vi "Func-엑셀 데이터를 그래프로 출력.vi"() -> ()   [LabVIEW 2015] (continued)
\n1158.26\n1158.28\n1158.3\n1158.31\n1158.33\n1158.34\n1158.36\n1158.38\n1158.39\n1158.41\n1158.43\n1158.44\n1158.46\n1158.48\n1158.49\n1158.51\n1158.53\n1158.55\n1158.56\n1158.58\n1158.59\n1158.61\n1158.63\n1158.65\n1158.66\n1158.68\n1158.69\n1158.71\n1158.73\n1158.74\n1158.76\n1158.78\n1158.8\n1158.81\n1158.83\n1158.84\n1158.86\n1158.88\n1158.89\n1158.91\n1158.93\n1158.94\n1158.96\n1158.98\n1159\n1159.01\n1159.03\n1159.04\n1159.06\n1159.08\n1159.09\n1159.11\n1159.13\n1159.15\n1159.16\n1159.18\n1159.19\n1159.21\n1159.23\n1159.25\n1159.26\n1159.28\n1159.29\n1159.31\n1159.33\n1159.35\n1159.36\n1159.38\n1159.39\n1159.41\n1159.43\n1159.44\n1159.46\n1159.48\n1159.5\n1159.51\n1159.53\n1159.54\n1159.56\n1159.58\n1159.59\n1159.61\n1159.63\n1159.64\n1159.66\n1159.68\n1159.69\n1159.71\n1159.73\n1159.74\n1159.76\n1159.78\n1159.79\n1159.81\n1159.83\n1159.84\n1159.86\n1159.88\n1159.89\n1159.91\n1159.93\n1159.94\n1159.96\n1159.98\n1159.99\n1160.01\n1160.03\n1160.04\n1160.06\n1160.08\n1160.09\n1160.11\n1160.13\n1160.14\n1160.16\n1160.18\n1160.19\n1160.21\n1160.23\n1160.24\n1160.26\n1160.28\n1160.29\n1160.31\n1160.33\n1160.34\n1160.36\n1160.38\n1160.39\n1160.41\n1160.43\n1160.44\n1160.46\n1160.48\n1160.49\n1160.51\n1160.53\n1160.54\n1160.56\n1160.58\n1160.59\n1160.61\n1160.63\n1160.64\n1160.66\n1160.68\n1160.69\n1160.71\n1160.73\n1160.74\n1160.76\n1160.78\n1160.79\n1160.81\n1160.83\n1160.84\n1160.86\n1160.88\n1160.89\n1160.91\n1160.93\n1160.94\n1160.96\n1160.98\n1160.99\n1161.01\n1161.03\n1161.04\n1161.06\n1161.08\n1161.09\n1161.11\n1161.13\n1161.14\n1161.16\n1161.18\n1161.19\n1161.21\n1161.23\n1161.24\n1161.26\n1161.28\n1161.3\n1161.31\n1161.33\n1161.34\n1161.36\n1161.38\n1161.39\n1161.41\n1161.43\n1161.44\n1161.46\n1161.48\n1161.49\n1161.51\n1161.53\n1161.55\n1161.56\n1161.58\n1161.59\n1161.61\n1161.63\n1161.65\n1161.66\n1161.68\n1161.69\n1161.71\n1161.73\n1161.75\n1161.76\n1161.78\n1161.79\n1161.81\n1161.83\n1161.84\n1161.86\n1161.88\n1161.9\n1161.91\n1161.93\n1161.94\n1161.96\n1161.98\n1162\n1162.01\n1162.03\n1162.04\n1162.06\n1162.08\n1162.1\n1162.11\n1162.13\n1162.14\n1162.16\n1162.18\n1162.19\n1162.21\n1162.23\n1162.25\n1162.26\n1162.28\n1162.29\n1162.31\n1162.33\n1162.35\n1162.36\n1162.38\n1162.39\n1162.41\n1162.43\n1162.45\n1162.46\n1162.48\n1162.49\n1162.51\n1162.53\n1162.55\n1162.56\n1162.58\n1162.59\n1162.61\n1162.63\n1162.64\n1162.66\n1162.68\n1162.7\n1162.71\n1162.73\n1162.74\n1162.76\n1162.78\n1162.79\n1162.81\n1162.83\n1162.84\n1162.86\n1162.88\n1162.89\n1162.91\n1162.93\n1162.95\n1162.96\n1162.98\n1162.99\n1163.01\n1180.53\n1180.71\n1180.87\n1181.04\n1181.21\n1181.37\n1181.55\n1181.71\n1181.88\n1182.05\n1182.21\n1182.38\n1182.55\n1182.71\n1182.88\n1183.05\n1183.21\n1183.38\n1183.55\n1183.72\n1183.88\n1184.05\n1184.21\n1184.38\n1184.55\n1184.71\n1184.88\n1185.05\n1185.21\n1185.38\n1185.55\n1185.71\n1185.88\n1186.06\n1186.22\n1186.39\n1186.56\n1186.73\n1186.9\n1187.07\n1187.23\n1187.4\n1187.56\n1187.73\n1187.9\n1188.06\n1188.23\n1188.4\n1188.56\n1188.73\n1188.9\n1189.07\n1189.24\n1189.41\n1189.57\n1189.74\n1189.91\n1190.07\n1190.24\n1190.41\n1190.57\n1190.74\n1190.91\n1191.07\n1191.24\n1191.41\n1191.57\n1191.74\n1191.91\n1192.07\n1192.24\n1192.41\n1192.57\n1192.74\n1192.91\n1193.07\n1193.24\n1193.41\n1193.57\n1193.74\n1193.91\n1194.07\n1194.24\n1194.41\n1194.57\n1194.74\n1194.91\n1195.07\n1195.24\n1195.41\n1195.57\n1195.74\n1195.91\n1196.07\n1196.24\n1196.41\n1196.57\n1196.74\n1196.91\n1197.07\n1197.24\n1197.41\n1197.58\n1197.75\n1197.91\n1198.08\n1198.25\n1198.42\n1198.58\n1198.75\n1198.91\n1199.08\n1199.25\n1199.41\n1199.58\n1199.75\n1199.91\n1200.08\n1200.25\n1200.41\n1200.58\n1200.75\n1200.91\n1201.08\n1201.25\n1201.42\n1201.58\n1201.75\n1201.92\n1202.09\n1202.26\n1202.42\n1202.59\n1202.76\n1202.92\n1203.09\n1203.26\n1203.42\n1203.6\n1203.76\n1203.93\n1204.1\n1204.27\n1204.43\n1204.6\n1204.77\n1204.93\n1205.1\n1205.26\n1205.43\n1205.6\n1205.76\n1205.93\n1206.1\n1206.26\n1206.43\n1206.6\n1206.76\n1206.93\n1207.1\n1207.26\n1207.43\n1207.6\n1207.76\n1207.93\n1208.1\n1208.26\n1208.43\n1208.6\n1208.76\n1208.93\n1209.1\n1209.26\n1209.43\n1209.6\n1209.76\n1209.93\n1210.1\n1210.26\n1210.43\n1210.6\n1210.76\n1210.93\n1211.1\n1211.26\n1211.43\n1211.6\n1211.76\n1211.93\n1212.11\n1212.28\n1212.45\n1212.61\n1212.78\n1212.95\n1213.12\n1213.28\n1213.45\n1213.61\n1213.78\n1213.95\n1214.11\n1214.28\n1214.45\n1214.61\n1214.79\n1214.96\n1215.12\n1215.29\n1215.46\n1215.62\n1215.79\n1215.96\n1216.12\n1216.29\n1216.46\n1216.62\n1216.79\n1216.96\n1217.13\n1217.3\n1217.47\n1217.64\n1217.81\n1217.97\n1218.14\n1218.31\n1218.48\n1218.65\n1218.81\n1218.98\n1219.15\n1219.32\n1219.48\n1219.65\n1219.81\n1219.98\n1220.15\n1220.31\n1220.48\n1220.65\n1220.81\n1220.99\n1221.17\n1221.33\n1221.5\n1221.66\n1221.83\n1222.01\n1222.18\n1222.35\n1222.51\n1222.68\n1222.85\n1223.02\n1223.18\n1223.35\n1223.51\n1223.68\n1223.85\n1224.01\n1224.17\n1224.18\n1224.19\n1224.21\n1224.23\n1224.24\n1224.26\n1224.28\n1224.29\n1224.31\n1224.33\n1224.34\n1224.36\n1224.38\n1224.39\n1224.41\n1224.43\n1224.44\n1224.46\n1224.48\n1224.49\n1224.51\n1224.53\n1224.54\n1224.56\n1224.58\n1224.59\n1224.61\n1224.63\n1224.64\n1224.66\n1224.68\n1224.69\n1224.71\n1224.73\n1224.74\n1224.76\n1224.78\n1224.79\n1224.81\n1224.83\n1224.84\n1224.86\n1224.88\n1224.89\n1224.91\n1224.93\n1224.94\n1224.96\n1224.98\n1224.99\n1225.01\n1225.03\n1225.05\n1225.06\n1225.08\n1225.09\n1225.11\n1225.13\n1225.14\n1225.16\n1225.18\n1225.19\n1225.21\n1225.23\n1225.24\n1225.26\n1225.28\n1225.29\n1225.31\n1225.33\n1225.34\n1225.36\n1225.38\n1225.39\n1225.41\n1225.43\n1225.44\n1225.46\n1225.48\n1225.49\n1225.51\n1225.53\n1225.54\n1225.56\n1225.58\n1225.59\n1225.61\n1225.63\n1225.64\n1225.66\n1225.68\n1225.69\n1225.71\n1225.73\n1225.74\n1225.76\n1225.78\n1225.79\n1225.81\n1225.83\n1225.85\n1225.86\n1225.88\n1225.89\n1225.91\n1225.93\n1225.94\n1225.96\n1225.98\n1225.99\n1226.01\n1226.03\n1226.04\n1226.06\n1226.08\n1226.1\n1226.11\n1226.13\n1226.14\n1226.16\n1226.18\n1226.2\n1226.21\n1226.23\n1226.25\n1226.26\n1226.28\n1226.3\n1226.31\n1226.33\n1226.34\n1226.36\n1226.38\n1226.39\n1226.41\n1226.43\n1226.44\n1226.46\n1226.48\n1226.49\n1226.51\n1226.53\n1226.55\n1226.56\n1226.58\n1226.59\n1226.61\n1226.63\n1226.64\n1226.66\n1226.68\n1226.7\n1226.71\n1226.73\n1226.74\n1226.76\n1226.78\n1226.79\n1226.81\n1226.83\n1226.84\n1226.86\n1226.88\n1226.9\n1226.91\n1226.93\n1226.94\n1226.96\n1226.98\n1226.99\n1227.01\n1227.03\n1227.04\n1227.06\n1227.08\n1227.09\n1227.11\n1227.13\n1227.14\n1227.16\n1227.18\n1227.19\n1227.21\n1227.23\n1227.24\n1227.26\n1227.28\n1227.29\n1227.31\n1227.33\n1227.34\n1227.36\n1227.38\n1227.4\n1227.41\n1227.43\n1227.44\n1227.46\n1227.48\n1227.49\n1227.51\n1227.53\n1227.54\n1227.56\n1227.58\n1227.59\n1227.61\n1227.63\n1227.64\n1227.66\n1227.68\n1227.69\n1227.71\n1227.73\n1227.74\n1227.76\n1227.78\n1227.8\n1227.81\n1227.83\n1227.84\n1227.86\n1227.88\n1227.89\n1227.91\n1227.93\n1227.94\n1227.96\n1227.98\n1227.99\n1228.01\n1228.03\n1228.04\n1228.06\n1228.08\n1228.09\n1228.11\n1228.13\n1228.14\n1228.16\n1228.18\n1228.19\n1228.21\n1228.23\n1228.24\n1228.26\n1228.28\n1228.29\n1228.31\n1228.33\n1228.34\n1228.36\n1228.38\n1228.39\n1228.41\n1228.43\n1228.44\n1228.46\n1228.48\n1228.49\n1228.51\n1228.53\n1228.54\n1228.56\n1228.58\n1228.6\n1228.61\n1228.63\n1228.64\n1228.66\n1228.68\n1228.69\n1228.71\n1228.73\n1228.74\n1228.76\n1228.78\n1228.79\n1228.81\n1228.83\n1228.85\n1228.86\n1228.88\n1228.89\n1228.91\n1228.93\n1228.95\n1228.96\n1228.98\n1229\n1229.01\n1229.03\n1229.04\n1229.06\n1229.08\n1229.09\n1229.11\n1229.13\n1229.14\n1229.16\n1229.18\n1229.2\n1229.21\n1229.23\n1229.24\n1229.26\n1229.28\n1229.3\n1229.31\n1229.33\n1229.34\n1229.36\n1229.38\n1229.4\n1229.41\n1229.43\n1229.44\n1229.46\n1229.48\n1229.49\n1229.51\n1229.53\n1229.55\n1229.56\n1229.58\n1229.59\n1229.61\n1229.63\n1229.64\n1229.66\n1229.68\n1229.69\n1229.71\n1229.73\n1229.74\n1229.76\n1229.78\n1229.79\n1229.81\n1229.83\n1229.84\n1229.86\n1229.88\n1229.89\n1229.91\n1229.93\n1229.94\n1229.96\n1229.98\n1229.99\n1230.01\n1230.03\n1230.04\n1230.06\n1230.08\n1230.09\n1230.11\n1230.13\n1230.14\n1230.16\n1230.18\n1230.19\n1230.21\n1230.23\n1230.24\n1230.26\n1230.28\n1230.29\n1230.31\n1230.33\n1230.34\n1230.36\n1230.38\n1230.39\n1230.41\n1230.43\n1230.44\n1230.46\n1230.48\n1230.49\n1230.51\n1230.53\n1230.54\n1230.56\n1230.58\n1230.59\n1230.61\n1230.63\n1230.64\n1230.66\n1230.68\n1230.69\n1230.71\n1230.73\n1230.74\n1230.76\n1230.78\n1230.79\n1230.81\n1230.83\n1230.84\n1230.86\n1230.88\n1230.89\n1230.91\n1230.93\n1230.94\n1230.96\n1230.98\n1230.99\n1231.01\n1231.03\n1231.04\n1231.06\n1231.08\n1231.09\n1231.11\n1231.13\n1231.14\n1231.16\n1231.18\n1231.19\n1231.21\n1231.23\n1231.24\n1231.26\n1231.28\n1231.29\n1231.31\n1231.33\n1231.34\n1231.36\n1231.38\n1231.39\n1231.41\n1231.43\n1231.44\n1231.46\n1231.48\n1231.49\n1231.51\n1231.53\n1231.54\n1231.56\n1231.58\n1231.6\n1231.61\n1231.63\n1231.64\n1231.66\n1231.68\n1231.69\n1231.71\n1231.73\n1231.74\n1231.76\n1231.78\n1231.79\n1231.81\n1231.83\n1231.84\n1231.86\n1231.88\n1231.89\n1231.91\n1231.93\n1231.95\n1231.96\n1231.98\n1231.99\n1232.01\n1232.03\n1232.05\n1232.06\n1232.08\n1232.09\n1232.11\n1232.13\n1232.14\n1232.16\n1232.18\n1232.2\n1232.21\n1232.23\n1232.24\n1232.26\n1232.28\n1232.3\n1232.31\n1232.33\n1232.34\n1232.36\n1232.38\n1232.4\n1232.41\n1232.43\n1232.44\n1232.46\n1232.48\n1232.49\n1232.51\n1232.53\n1232.54\n1232.56\n1232.58\n1232.59\n1232.61\n1232.63\n1232.64\n1232.66\n1232.68\n1232.69\n1232.71\n1232.73\n1232.74\n1232.76\n1232.78\n1232.79\n1232.81\n1232.83\n1232.84\n1232.86\n1232.88\n1232.89\n1232.91\n1232.93\n1232.94\n1232.96\n1232.98\n1232.99\n1233.01\n1233.03\n1233.04\n1233.06\n1233.08\n1233.09\n1233.11\n1233.13\n1233.14\n1233.16\n1233.18\n1233.19\n1233.21\n1233.23\n1233.24\n1233.26\n1233.28\n1233.29\n1233.31\n1233.33\n1233.34\n1233.36\n1233.38\n1233.39\n1233.41\n1233.43\n1233.44\n1233.46\n1233.48\n1233.49\n1233.51\n1233.53\n1233.54\n1233.56\n1233.58\n1233.59\n1233.61\n1233.63\n1233.64\n1233.66\n1233.68\n1233.69\n1233.71\n1233.73\n1233.74\n1233.76\n1233.78\n1233.79\n1233.81\n1233.83\n1233.84\n1233.86\n1233.88\n1233.89\n1233.91\n1233.93\n1233.94\n1233.96\n1233.98\n1233.99\n1234.01\n1234.03\n1234.04\n1234.06\n1234.08\n1234.09\n1234.11\n1234.13\n1234.14\n1234.16\n1234.18\n1234.19\n1234.21\n1234.23\n1234.24\n1234.26\n1234.28\n1234.29\n1234.31\n1234.33\n1234.35\n1234.36\n1234.38\n1234.39\n1234.41\n1234.43\n1234.44\n1234.46\n1234.48\n1234.49\n1234.51\n1234.53\n1234.54\n1234.56\n1234.58\n1234.59\n1234.61\n1234.63\n1234.64\n1234.66\n1234.68\n1234.7\n1234.71\n1234.73\n1234.74\n1234.76\n1234.78\n1234.8\n1234.81\n1234.83\n1234.84\n1234.86\n1234.88\n1234.89\n1234.91\n1234.93\n1234.95\n1234.96\n1234.98\n1234.99\n1235.01\n1235.03\n1235.05\n1235.06\n1235.08\n1235.09\n1235.11\n1235.13\n1235.15\n1235.16\n1235.18\n1235.19\n1235.21\n1235.23\n1235.24\n1235.26\n1235.28\n1235.3\n1235.31\n1235.33\n1235.34\n1235.36\n1235.38\n1235.39\n1235.41\n1235.43\n1235.44\n1235.46\n1235.48\n1235.5\n1235.51\n1235.53\n1235.54\n1235.56\n1235.58\n1235.59\n1235.61\n1235.63\n1235.65\n1235.66\n1235.68\n1235.69\n1235.71\n1235.73\n1235.74\n1235.76\n1235.78\n1235.79\n1235.81\n1235.83\n1235.85\n1235.86\n1235.88\n1235.89\n1235.91\n1235.93\n1235.94\n1235.96\n1235.98\n1235.99\n1236.01\n1236.03\n1236.04\n1236.06\n1236.08\n1236.09\n1236.11\n1236.13\n1236.14\n1236.16\n1236.18\n1236.19\n1236.21\n1236.23\n1236.24\n1236.26\n1236.28\n1236.29\n1236.31\n1236.33\n1236.34\n1236.36\n1236.38\n1236.39\n1236.41\n1236.43\n1236.44\n1236.46\n1236.48\n1236.49\n1236.51\n1236.53\n1236.54\n1236.56\n1236.58\n1236.59\n1236.61\n1236.63\n1236.64\n1236.66\n1236.68\n1236.69\n1236.71\n1236.73\n1236.74\n1236.76\n1236.78\n1236.79\n1236.81\n1236.83\n1236.84\n1236.86\n1236.88\n1236.89\n1236.91\n1236.93\n1236.94\n1236.96\n1236.98\n1236.99\n1237.01\n1237.03\n1237.04\n1237.06\n1237.08\n1237.09\n1237.11\n1237.13\n1237.14\n1237.16\n1237.18\n1237.19\n1237.21\n1237.23\n1237.24\n1237.26\n1237.28\n1237.29\n1237.31\n1237.33\n1237.34\n1237.36\n1237.38\n1237.39\n1237.41\n1237.43\n1237.44\n1237.46\n1237.48\n1237.49\n1237.51\n1237.53\n1237.54\n1237.56\n1237.58\n1237.59\n1237.61\n1237.63\n1237.64\n1237.66\n1237.68\n1237.7\n1237.71\n1237.73\n1237.74\n1237.76\n1237.78\n1237.8\n1237.81\n1237.83\n1237.84\n1237.86\n1237.88\n1237.89\n1237.91\n1237.93\n1237.94\n1237.96\n1237.98\n1237.99\n1238.01\n1238.03\n1238.04\n1238.06\n1238.08\n1238.09\n1238.11\n1238.13\n1238.15\n1238.16\n1238.18\n1238.2\n1238.21\n1238.23\n1238.24\n1238.26\n1238.28\n1238.29\n1238.31\n1238.33\n1238.34\n1238.36\n1238.38\n1238.39\n1238.41\n1238.43\n1238.44\n1238.46\n1238.48\n1238.5\n1238.51\n1238.53\n1238.54\n1238.56\n1238.58\n1238.6\n1238.61\n1238.63\n1238.64\n1238.66\n1238.68\n1238.69\n1238.71\n1238.73\n1238.74\n1238.76\n1238.78\n1238.79\n1238.81\n1238.83\n1238.84\n1238.86\n1238.88\n1238.89\n1238.91\n1238.93\n1238.94\n1238.96\n1238.98\n1238.99\n1239.01\n1239.03\n1239.04\n1239.06\n1239.08\n1239.09\n1239.11\n1239.13\n1239.14\n1239.16\n1239.18\n1239.19\n1239.21\n1239.23\n1239.24\n1239.26\n1239.28\n1239.29\n1239.31\n1239.33\n1239.34\n1239.36\n1239.38\n1239.39\n1239.41\n1239.43\n1239.44\n1239.46\n1239.48\n1239.49\n1239.51\n1239.53\n1239.54\n1239.56\n1239.58\n1239.59\n1239.61\n1239.63\n1239.64\n1239.66\n1239.68\n1239.69\n1239.71\n1239.73\n1239.74\n1239.76\n1239.78\n1239.79\n1239.81\n1239.83\n1239.84\n1239.86\n1239.88\n1239.89\n1239.91\n1239.93\n1239.94\n1239.96\n1239.98\n1239.99\n1240.01\n1240.03\n1240.04\n1240.06\n1240.08\n1240.09\n1240.11\n1240.13\n1240.14\n1240.16\n1240.18\n1240.19\n1240.21\n1240.23\n1240.24\n1240.26\n1240.28\n1240.29\n1240.31\n1240.33\n1240.34\n1240.36\n1240.38\n1240.39\n1240.41\n1240.43\n1240.44\n1240.46\n1240.48\n1240.49\n1240.51\n1240.53\n1240.55\n1240.56\n1240.58\n1240.59\n1240.61\n1240.63\n1240.64\n1240.66\n1240.68\n1240.69\n1240.71\n1240.73\n1240.74\n1240.76\n1240.78\n1240.79\n1240.81\n1240.83\n1240.84\n1240.86\n1240.88\n1240.9\n1240.91\n1240.93\n1240.94\n1240.96\n1240.98\n1240.99\n1241.01\n1241.03\n1241.05\n1241.06\n1241.08\n1241.09\n1241.11\n1241.13\n1241.15\n1241.16\n1241.18\n1241.19\n1241.21\n1241.23\n1241.25\n1241.26\n1241.28\n1241.29\n1241.31\n1241.33\n1241.35\n1241.36\n1241.38\n1241.39\n1241.41\n1241.43\n1241.44\n1241.46\n1241.48\n1241.5\n1241.51\n1241.53\n1241.54\n1241.56\n1241.58\n1241.6\n1241.61\n1241.63\n1241.64\n1241.66\n1241.68\n1241.69\n1241.71\n1241.73\n1241.74\n1241.76\n1241.78\n1241.79\n1241.81\n1241.83\n1241.84\n1241.86\n1241.88\n1241.89\n1241.91\n1241.93\n1241.94\n1241.96\n1241.98\n1242\n1242.01\n1242.03\n1242.04\n1242.06\n1242.08\n1242.1\n1242.11\n1242.13\n1242.14\n1242.16\n1242.18\n1242.19\n1242.21\n1242.23\n1242.24\n1242.26\n1242.28\n1242.29\n1242.31\n1242.33\n1242.34\n1242.36\n1242.38\n1242.39\n1242.41\n1242.43\n1242.44\n1242.46\n1242.48\n1242.49\n1242.51\n1242.53\n1242.54\n1242.56\n1242.58\n1242.59\n1242.61\n1242.63\n1242.64\n1242.66\n1242.68\n1242.69\n1242.71\n1242.73\n1242.74\n1242.76\n1242.78\n1242.79\n1242.81\n1242.83\n1242.84\n1242.86\n1242.88\n1242.89\n1242.91\n1242.93\n1242.94\n1242.96\n1242.98\n1242.99\n1243.01\n1243.03\n1243.04\n1243.06\n1243.08\n1243.09\n1243.11\n1243.13\n1243.14\n1243.16\n1243.18\n1243.19\n1243.21\n1243.23\n1243.24\n1243.26\n1243.28\n1243.29\n1243.31\n1243.33\n1243.34\n1243.36\n1243.38\n1243.39\n1243.41\n1243.43\n1243.45\n1243.46\n1243.48\n1243.49\n1243.51\n1243.53\n1243.54\n1243.56\n1243.58\n1243.59\n1243.61\n1243.63\n1243.65\n1243.66\n1243.68\n1243.69\n1243.71\n1243.73\n1243.74\n1243.76\n1243.78\n1243.79\n1243.81\n1243.83\n1243.84\n1243.86\n1243.88\n1243.9\n1243.91\n1243.93\n1243.94\n1243.96\n1243.98\n1244\n1244.01\n1244.03\n1244.04\n1244.06\n1244.08\n1244.09\n1244.11\n1244.13\n1244.14\n1244.16\n1244.18\n1244.19\n1244.21\n1244.23\n1244.25\n1244.26\n1244.28\n1244.29\n1244.31\n1244.33\n1244.35\n1244.36\n1244.38\n1244.4\n1244.41\n1244.43\n1244.44\n1244.46\n1244.48\n1244.49\n1244.51\n1244.53\n1244.54\n1244.56\n1244.58\n1244.6\n1244.61\n1244.63\n1244.64\n1244.66\n1244.68\n1244.69\n1244.71\n1244.73\n1244.74\n1244.76\n1244.78\n1244.79\n1244.81\n1244.83\n1244.84\n1244.86\n1244.88\n1244.89\n1244.91\n1244.93\n1244.94\n1244.96\n1244.98\n1244.99\n1245.01\n1245.03\n1245.04\n1245.06\n1245.08\n1245.09\n1245.11\n1245.13\n1245.14\n1245.16\n1245.18\n1245.19\n1245.21\n1245.23\n1245.24\n1245.26\n1245.28\n1245.29\n1245.31\n1245.33\n1245.34\n1245.36\n1245.38\n1245.39\n1245.41\n1245.43\n1245.44\n1245.46\n1245.48\n1245.49\n1245.51\n1245.53\n1245.54\n1245.56\n1245.58\n1245.59\n1245.61\n1245.63\n1245.64\n1245.66\n1245.68\n1245.69\n1245.71\n1245.73\n1245.74\n1245.76\n1245.78\n1245.79\n1245.81\n1245.83\n1245.85\n1245.86\n1245.88\n1245.89\n1245.91\n1245.93\n1245.94\n1245.96\n1245.98\n1245.99\n1246.01\n1246.03\n1246.04\n1246.06\n1246.08\n1246.09\n1246.11\n1246.13\n1246.14\n1246.16\n1246.18\n1246.19\n1246.21\n1246.23\n1246.24\n1246.26\n1246.28\n1246.29\n1246.31\n1246.33\n1246.34\n1246.36\n1246.38\n1246.39\n1246.41\n1246.43\n1246.44\n1246.46\n1246.48\n1246.49\n1246.51\n1246.53\n1246.54\n1246.56\n1246.58\n1246.59\n1246.61\n1246.63\n1246.64\n1246.66\n1246.68\n1246.69\n1246.71\n1246.73\n1246.74\n1246.76\n1246.78\n1246.8\n1246.81\n1246.83\n1246.84\n1246.86\n1246.88\n1246.89\n1246.91\n1246.93\n1246.94\n1246.96\n1246.98\n1246.99\n1247.01\n1247.03\n1247.04\n1247.06\n1247.08\n1247.1\n1247.11\n1247.13\n1247.14\n1247.16\n1247.18\n1247.19\n1247.21\n1247.23\n1247.24\n1247.26\n1247.28\n1247.29\n1247.31\n1247.33\n1247.35\n1247.36\n1247.38\n1247.39\n1247.41\n1247.43\n1247.45\n1247.46\n1247.48\n1247.49\n1247.51\n1247.53\n1247.55\n1247.56\n1247.58\n1247.6\n1247.61\n1247.63\n1247.64\n1247.66\n1247.68\n1247.69\n1247.71\n1247.73\n1247.74\n1247.76\n1247.78\n1247.8\n1247.81\n1247.83\n1247.84\n1247.86\n1247.88\n1247.9\n1247.91\n1247.93\n1247.95\n1247.96\n1247.98\n1247.99\n1248.01\n1248.03\n1248.05\n1248.06\n1248.08\n1248.09\n1248.11\n1248.13\n1248.14\n1248.16\n1248.18\n1248.19\n1248.21\n1248.23\n1248.24\n1248.26\n1248.28\n1248.29\n1248.31\n1248.33\n1248.34\n1248.36\n1248.38\n1248.39\n1248.41\n1248.43\n1248.44\n1248.46\n1248.48\n1248.49\n1248.51\n1248.53\n1248.54\n1248.56\n1248.58\n1248.59\n1248.61\n1248.63\n1248.64\n1248.66\n1248.68\n1248.69\n1248.71\n1248.73\n1248.74\n1248.76\n1248.78\n1248.79\n1248.81\n1248.83\n1248.84\n1248.86\n1248.88\n1248.89\n1248.91\n1248.93\n1248.94\n1248.96\n1248.98\n1248.99\n1249.01\n1249.03\n1249.05\n1249.06\n1249.08\n1249.09\n1249.11\n1249.13\n1249.14\n1249.16\n1249.18\n1249.19\n1249.21\n1249.23\n1249.24\n1249.26\n1249.28\n1249.29\n1249.31\n1249.33\n1249.34\n1249.36\n1249.38\n1249.39\n1249.41\n1249.43\n1249.44\n1249.46\n1249.48\n1249.49\n1249.51\n1249.53\n1249.54\n1249.56\n1249.58\n1249.59\n1249.61\n1249.63\n1249.64\n1249.66\n1249.68\n1249.69\n1249.71\n1249.73\n1249.74\n1249.76\n1249.78\n1249.79\n1249.81\n1249.83\n1249.85\n1249.86\n1249.88\n1249.89\n1249.91\n1249.93\n1249.94\n1249.96\n1249.98\n1250\n1250.01\n1250.03\n1250.04\n1250.06\n1250.08\n1250.1\n1250.11\n1250.13\n1250.14\n1250.16\n1250.18\n1250.2\n1250.21\n1250.23\n1250.24\n1250.26\n1250.28\n1250.29\n1250.31\n1250.33\n1250.34\n1250.36\n1250.38\n1250.39\n1250.41\n1250.43\n1250.45\n1250.46\n1250.48\n1250.5\n1250.51\n1250.53\n1250.55\n1250.56\n1250.58\n1250.59\n1250.61\n1250.63\n1250.64\n1250.66\n1250.68\n1250.7\n1250.71\n1250.73\n1250.74\n1250.76\n1250.78\n1250.8\n1250.81\n1250.83\n1250.84\n1250.86\n1250.88\n1250.89\n1250.91\n1250.93\n1250.95\n1250.96\n1250.98\n1250.99\n1251.01\n1251.03\n1251.04\n1251.06\n1251.08\n1251.09\n1251.11\n1251.13\n1251.14\n1251.16\n1251.18\n1251.19\n1251.21\n1251.23\n1251.25\n1251.26\n1251.28\n1251.29\n1251.31\n1251.33\n1251.34\n1251.36\n1251.38\n1251.39\n1251.41\n1251.43\n1251.44\n1251.46\n1251.48\n1251.5\n1251.51\n1251.53\n1251.54\n1251.56\n1251.58\n1251.59\n1251.61\n1251.63\n1251.64\n1251.66\n1251.68\n1251.69\n1251.71\n1251.73\n1251.74\n1251.76\n1251.78\n1251.79\n1251.81\n1251.83\n1251.84\n1251.86\n1251.88\n1251.89\n1251.91\n1251.93\n1251.94\n1251.96\n1251.98\n1251.99\n1252.01\n1252.03\n1252.04\n1252.06\n1252.08\n1252.09\n1252.11\n1252.13\n1252.14\n1252.16\n1252.18\n1252.19\n1252.21\n1252.23\n1252.24\n
